vi "findVISA-Port.vi"(10 "VISA list":refnum<visa-resource-name>[](array[refnum])=["ASRL1::INSTR", "NOEXIST", "ASRL3::INSTR", "NOEXIST", "NOEXIST", "NOEXIST", "NOEXIST", "NOEXIST", "NOEXIST", "NOEXIST", "NOEXIST", "NOEXIST", "NOEXIST", "NOEXIST"], 11 "portNum":i32=1) -> (2 "matchFound":bool, 3 "found VISA":refnum<visa-resource-name>)   [LabVIEW 2012]
doc: "find the match one for portNum from available ASRL, this PortNum = COM Number during NportAdmin setup \n\nmatchfound=T or F"
panel:
  out "loop":i32
  out "search":string
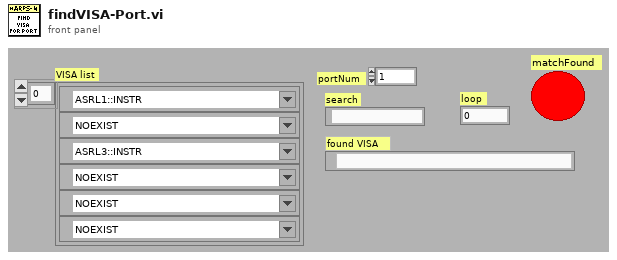
[diagram p1: front panel]
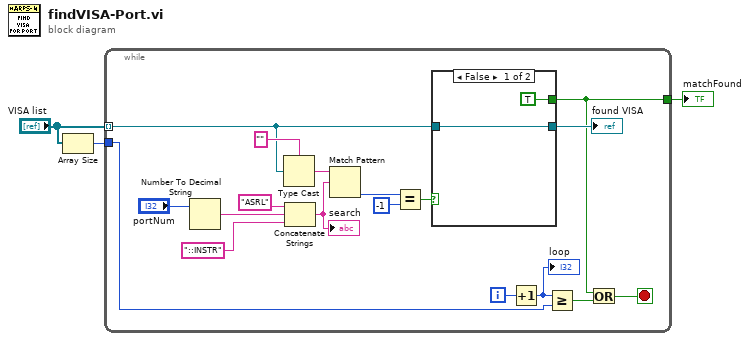
[diagram p0: block diagram]
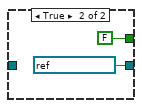
[diagram p2: hidden frame]
diagram:
  n1 = Array Size(array="VISA list") -> (size(s)=w3:i32)
  n2 = while {
    tunnel: w3 -> [w10]
    tunnel: [w6] -> w2
    tunnel: "VISA list" -> [w5] mode=indexing
    i -> [w11]
    stop <- w7 stop-if-true
    n3 = Number To Decimal String(number="portNum") -> (decimal integer string=w20:string)  [unwired: 1 in]
    n4 = Type Cast(type="", x=w5) -> (*(type *) &x=w18:string)
    n5 = Concatenate Strings("ASRL" ("string"), w20, "::INSTR" ("string")) -> (w17:string)
    "search" <- w17
    n6 = Match Pattern(string=w18, regular expression=w17) -> (offset past match=w16:i32)  [unwired: 1 in, 3 out]
    n7 = Equal?(x=w16, y=-1) -> (x = y?=w14:bool)
    n8 = case shown="False" w14 {
      tunnel: [w22 refnum<visa-resource-name> "NOMATCH" ("found VISA  2")] -> w12
      tunnel: [TRUE FALSE] -> w6
      tunnel: w5 -> [w22 _]
      frame False {
      }
      frame True {
      }
    }
    "found VISA" <- w12
    n9 = Increment(x=w11) -> (x+1=w9:i32)
    "loop" <- w9
    n10 = Greater Or Equal?(x=w9, y=w10) -> (x >= y?=w8:bool)
    n11 = Or(x=w6, y=w8) -> (x .or. y?=w7:bool)
  }
  "matchFound" <- w2
